vi "add_group.vi"(0 "Experiments groups in":refnum<class "Experiments_group.lvclass">[](array[class]), 1 "Commentaires group":string="...write group description...", 3 "Name group":string, 5 "group":refnum<vi>, 7 "RadioButtonsControl":enum32{"Automatic", "User-def"}(ring), 9 "Folder path":path, 11 "error in (no error)":errorcluster, 12 "Upload":bool) -> (4 "Experiments groups out":refnum<class "Experiments_group.lvclass">[](array[class]), 15 "error out":errorcluster)   [LabVIEW 2015]
uses:
  Classes/Experiments/Experiments_group.lvclass
  Classes/Experiments/Experiment.lvclass
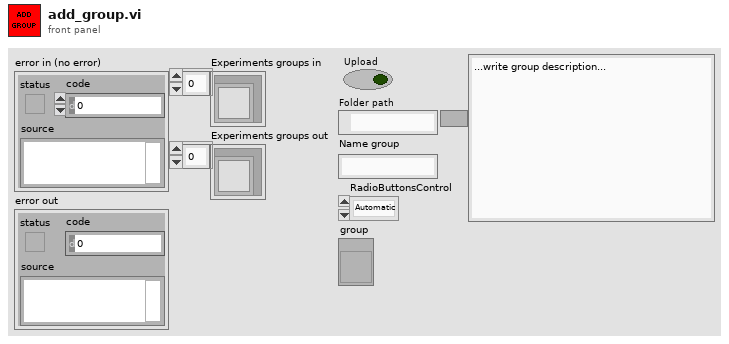
[diagram p1: front panel]
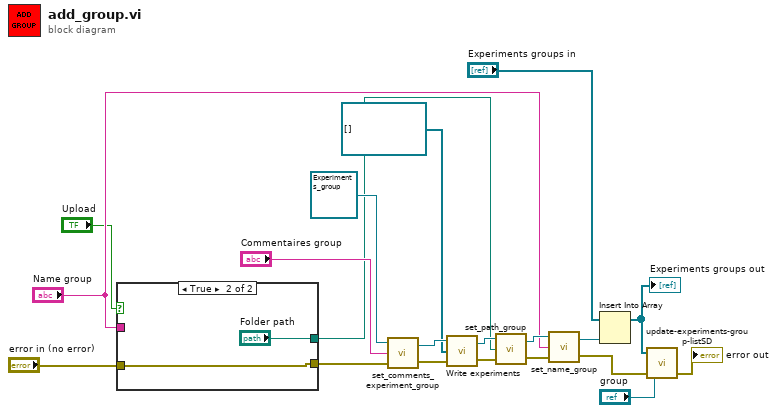
[diagram p0: block diagram]
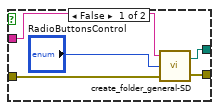
[diagram p2: hidden frame]
diagram:
  n1 = case shown="True" "Upload" {
    tunnel: [w24 w27] -> w15
    tunnel: "error in (no error)" -> [w23 w27]
    tunnel: [w22 "Folder path"] -> w3
    tunnel: "Name group" -> [w21 _]
    frame False {
      n2 = call "create_folder_general-SD.vi"("error in (no error)"=w23, "save Radio Buttons"="RadioButtonsControl", "Name"=w21) -> ("error out"=w24:errorcluster, "appended path"=w22:path)
    }
    frame True {
    }
  }
  n3 = call-dynamic "set_comments_experiment_group.vi"("error in (no error)"=w15, "Comments"="Commentaires group", "Experiments_group.lvclass in"=refnum<class "Experiments_group.lvclass"> refnum ("element")) -> ("error out"=w16:errorcluster, "Experiments_group.lvclass out"=w13:refnum<class "Experiments_group.lvclass">)
  n4 = call-dynamic "Write experiments.vi"("error in (no error)"=w16, "Experiments"=refnum<class "Experiment.lvclass">[] [] ("Experiment array"), "Experiments_group.lvclass in"=w13) -> ("error out"=w17:errorcluster, "Experiments_group.lvclass out"=w14:refnum<class "Experiments_group.lvclass">)
  n5 = call-dynamic "set_path_group.vi"("error in (no error)"=w17, "Path"=w3, "Experiments_group.lvclass in"=w14) -> ("error out"=w5:errorcluster, "Experiments_group.lvclass out"=w7:refnum<class "Experiments_group.lvclass">)
  n6 = call-dynamic "set_name_group.vi"("error in (no error)"=w5, "Name"="Name group", "Experiments_group.lvclass in"=w7) -> ("error out"=w4:errorcluster, "Experiments_group.lvclass out"=w6:refnum<class "Experiments_group.lvclass">)
  n7 = Insert Into Array(array="Experiments groups in", new element=w6) -> (w11:refnum<class "Experiments_group.lvclass">[])  [unwired: 1 in]
  "Experiments groups out" <- w11
  n8 = call "update-experiments-group-listSD.vi"("Experiments groups"=w11, "Group"="group", "error in (no error)"=w4) -> ("error out"=→"error out":errorcluster)  [unwired: 6 in]
